vi "get_edge_attribute.vi"(7 "attribute-name":string, 8 "error in (no error)":errorcluster, 9 "default value (empty variant)":variant, 10 "edge":refnum<class "Edge.lvclass">, 11 "graph":refnum<class "Graph.lvclass">) -> (0 "error out":errorcluster, 1 "attribute-value":variant, 2 "attribute-found":bool, 3 "graph-out":refnum<class "Graph.lvclass">)   [LabVIEW 2020, in "graph.lvlib" / "Graph.lvclass"]
uses:
  Graph.lvclass
  Graph.lvclass/Graph.ctl
  Edge/Edge.lvclass
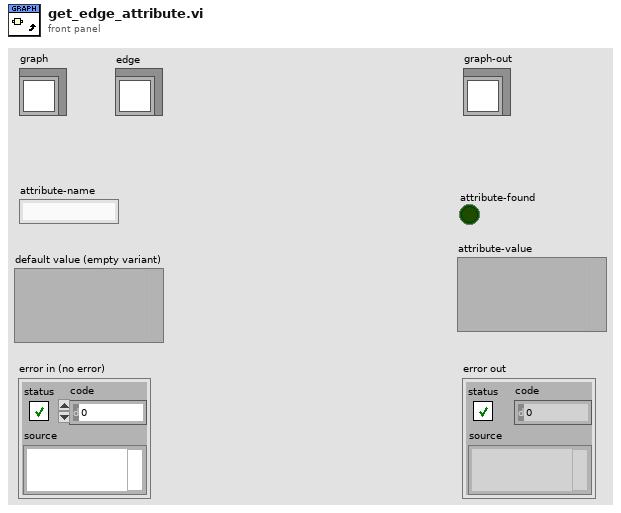
[diagram p1: front panel]
types:
  T1 = typedef "graph.lvlib/Graph.lvclass/edge-definition-cluster.ctl" = cluster{"source-id":refnum<class "ID.lvclass">, "sink-id":refnum<class "ID.lvclass">}
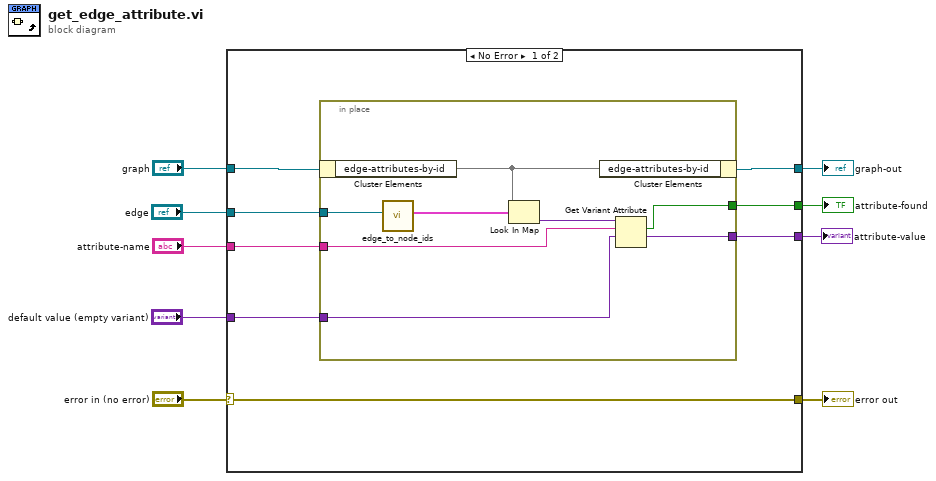
[diagram p0: block diagram]
diagram:
  n1 = case shown="No Error" "error in (no error)" {
    selector: "error in (no error)" -> [w17 w27]
    tunnel: [w17 w27] -> w8
    tunnel: [w15 w26] -> w6
    tunnel: "graph" -> [w14 w26]
    tunnel: "attribute-name" -> [w16 _]
    tunnel: "edge" -> [w13 _]
    tunnel: [w12 _] -> w3
    tunnel: "default value (empty variant)" -> [w11 _]
    tunnel: [w10 _] -> w1
    frame No Error {
      n2 = in-place {
        in-place-border: w16 -> [w23]
        in-place-border: w13 -> [w19]
        in-place-border: [w22] -> w12
        in-place-border: w11 -> [w21]
        in-place-border: [w20] -> w10
        n3 = in-place-cluster #1(w14) -> ("edge-attributes-by-id"=w25:map{T1, variant})
        n4 = call "edge_to_node_ids.vi"("edge"=w19) -> ("node-ids-cluster"=w18:T1)  [unwired: 10 in]
        n5 = Look In Map(map=w25, key=w18) -> (value=w24:variant)  [unwired: 1 in, 1 out]
        n6 = in-place-cluster #1("edge-attributes-by-id"=w25) -> (w15:refnum<class "Graph.lvclass">)
        n7 = Get Variant Attribute(Variant=w24, name=w23, default value (empty Variant)=w21) -> (found=w20:bool, value=w22:variant)  [unwired: 1 in, 2 out]
      }
    }
    frame Error {
    }
  }
  "error out" <- w8
  "graph-out" <- w6
  "attribute-value" <- w3
  "attribute-found" <- w1
